vi "destroy.vi"(8 "error in (no error)":errorcluster, 11 "system.logging.provider in":refnum<class "system.logging.provider.lvclass">) -> (0 "error out":errorcluster)   [LabVIEW 2021, in "system.logging.provider.lvclass"]
uses:
  system.logging.provider.lvclass
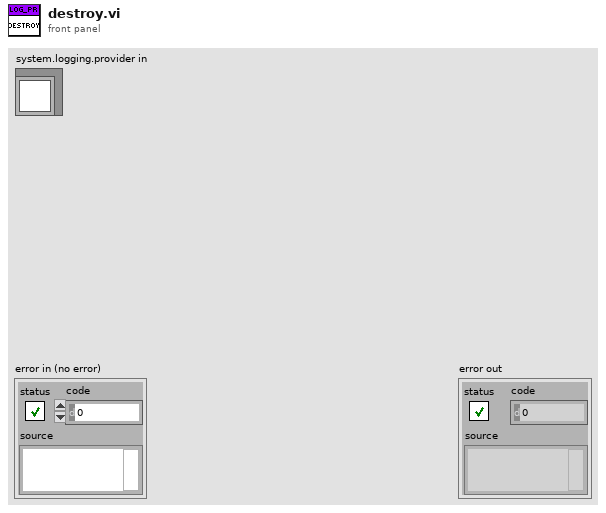
[diagram p1: front panel]
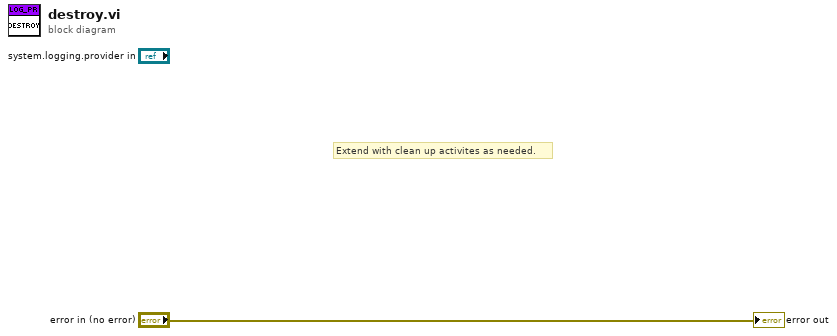
[diagram p0: block diagram]
diagram:
  # "Extend with clean up activites as needed."
  "error out" <- "error in (no error)"
